vi "Configure Controller Stable Response.vi"(8 "error in (no error)":errorcluster, 9 "stable response":u8=128, 10 "node address (same)":u8, 11 "ProPar in":refnum<class "PL Bronkhorst ProPar.lvclass">) -> (0 "error out":errorcluster, 3 "ProPar out":refnum<class "PL Bronkhorst ProPar.lvclass">)   [LabVIEW 2015, in "PL Bronkhorst ProPar.lvclass"]
doc: "Configures controller response when controller is stable (within 2% of the setpoint) of the specified <b>node</b>. Value 128 means no correction."
uses:
  PL Bronkhorst ProPar.lvclass
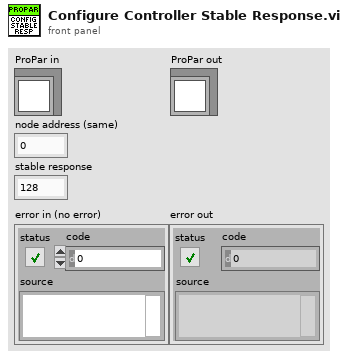
[diagram p1: front panel]
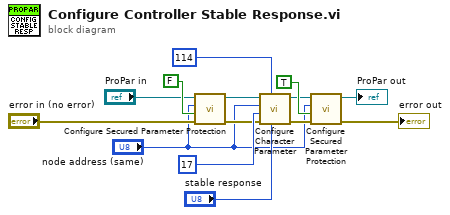
[diagram p0: block diagram]
diagram:
  n1 = call "Configure Secured Parameter Protection.vi"("error in (no error)"="error in (no error)", "enable protection"=FALSE, "node"="node address (same)", "ProPar in"="ProPar in") -> ("error out"=w7:errorcluster, "ProPar out"=w8:refnum<class "PL Bronkhorst ProPar.lvclass">)  [unwired: 6 in]
  n2 = call "Configure Character Parameter.vi"("value"="stable response", "process number"=u8 114, "error in (no error)"=w7, "parameter number"=u8 17 ("process number"), "node"="node address (same)", "ProPar in"=w8) -> ("error out"=w5:errorcluster, "ProPar out"=w2:refnum<class "PL Bronkhorst ProPar.lvclass">)  [unwired: 4 in]
  n3 = call "Configure Secured Parameter Protection.vi"("error in (no error)"=w5, "enable protection"=TRUE, "node"="node address (same)", "ProPar in"=w2) -> ("error out"=→"error out":errorcluster, "ProPar out"=→"ProPar out":refnum<class "PL Bronkhorst ProPar.lvclass">)  [unwired: 6 in]
